vi "Add packages to feed.vi"(0 "Feed Path":path, 5 "Packages Path":path, 11 "error in (no error)":errorcluster) -> (15 "error out":errorcluster)   [LabVIEW 2021, in "Packager Helpers.lvlib"]
uses:
  Packager Helpers.lvlib
  Path Functions/Path Functions.lvlib
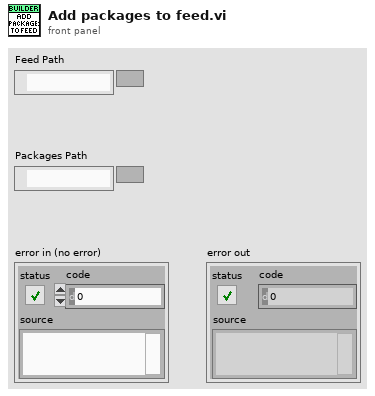
[diagram p1: front panel]
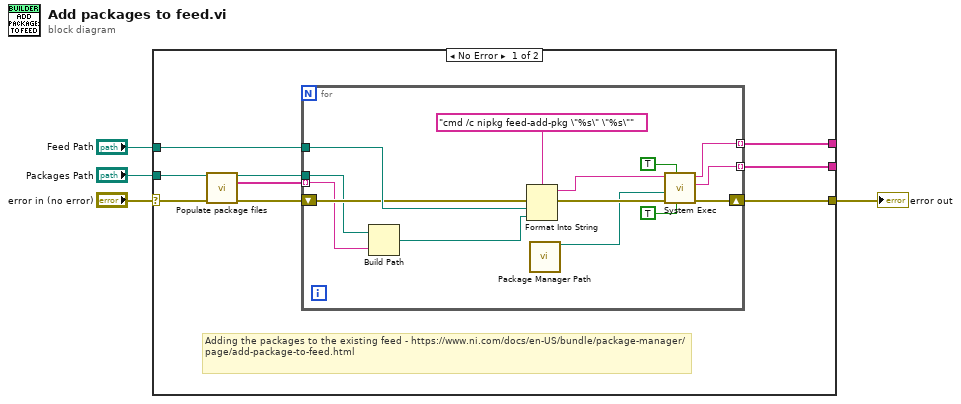
[diagram p0: block diagram]
diagram:
  n1 = case shown="No Error" "error in (no error)" {
    selector: "error in (no error)" -> [w9 w28]
    tunnel: [w13 w28] -> w3
    tunnel: "Feed Path" -> [w12 _]
    tunnel: "Packages Path" -> [w11 _]
    tunnel: [w6 _] -> _
    tunnel: [w5 _] -> _
    frame No Error {
      # "Adding the packages to the existing feed - https://www.ni.com/docs/en-US/bundle/package-manager/page/add-package-to-feed.html"
      n2 = call "Populate package files.vi"("Packages Path"=w11, "error in (no error)"=w9) -> ("path out"=w7:path, "filenames"=w8:string[], "error out"=w10:errorcluster)  [unwired: 11 in]
      n3 = for {
        tunnel: w12 -> [w20]
        shift-right: [w22] -> w13
        shift-left: w10 -> [w19]
        tunnel: w8 -> [w17] mode=indexing
        tunnel: w7 -> [w18]
        tunnel: [w15] -> w5 mode=indexing
        tunnel: [w14] -> w6 mode=indexing
        n4 = Build Path(base path=w18, name or relative path=w17) -> (appended path=w16:path)
        n5 = Format Into String(format string="cmd /c nipkg feed-add-pkg \"%s\" \"%s\"", error in=w19, w20, w16) -> (resulting string=w25:string, error out=w24:errorcluster)  [unwired: 1 in]
        n6 = call "Package Manager Path.vi"() -> ("Package Manager"=w21:path)  [unwired: 15 in]
        n7 = call <vilib>:"System Exec.vi"("run minimized? (F)"=TRUE, "wait until completion? (T)"=TRUE, "error in (no error)"=w24, "working directory"=w21, "command line"=w25) -> ("error out"=w22:errorcluster, "standard error"=w15:string, "standard output"=w14:string)  [unwired: 3 in, 1 out]
      }
    }
    frame Error {
    }
  }
  "error out" <- w3
